vi "changetoStaging.vi"(7 "cmd":enum16{"off", "on", "undulator", "staging"}(ring), 8 "error in (no error)":errorcluster, 10 "send (true)":bool=TRUE) -> (0 "error out":errorcluster)   [LabVIEW 2013]
panel:
  in  "curent set":u16
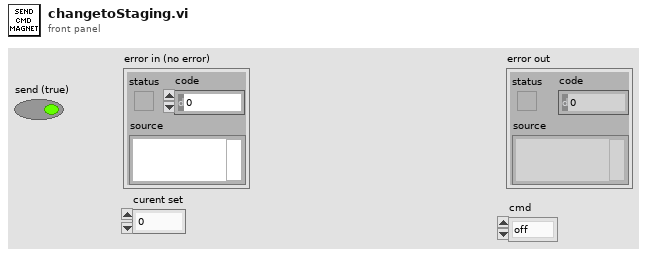
[diagram p1: front panel]
types:
  T1 = enum16{"Read", "Write", "ReadWrite", "BufferedRead", "BufferedReadWrite"}
  T2 = cluster{"data string":string, "data string":string, "data string":string, "data string":string}
  T3 = cluster{"match + rest of string":string, "match + rest of string":string, "data string":string, "data string":string}
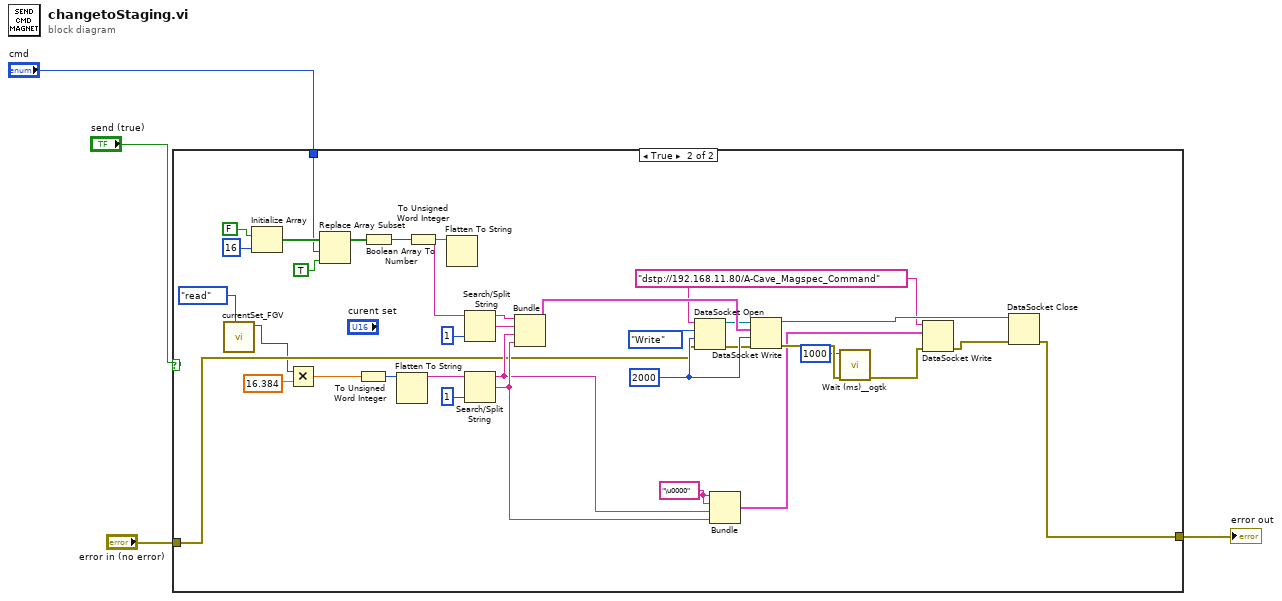
[diagram p0: block diagram]
diagram:
  n1 = case shown="True" "send (true)" {
    tunnel: "error in (no error)" -> [w5 w10]
    tunnel: [w5 w9] -> w2
    tunnel: "cmd" -> [_ w8]
    frame False {
    }
    frame True {
      w11 = "dstp://192.168.11.80/A-Cave_Magspec_Command" ("Target_URL")
      w21 = 2000 ("ms timeout (10000)")
      w22 = "\u0000" ("match + rest of string")
      n2 = call "currentSet_FGV.vi"("Enum"=enum16{"set", "read"}."read") -> ("curent set out"=w7:u16)  [unwired: 10 in]
      n3 = Initialize Array(FALSE, 16 ("dimension size")) -> (w39:bool[])
      n4 = Multiply(x=w7, y=16.384) -> (x*y=w28:dbl)
      n5 = Replace Array Subset(array=w39, new element=TRUE, index=w8) -> (w37:bool[])
      n6 = To Unsigned Word Integer(number=w28) -> (unsigned 16bit integer=w29:u16)
      n7 = Boolean Array To Number(Boolean array=w37) -> (number=w36:u32)
      n8 = Flatten To String(anything=w29) -> (data string=w30:string)  [unwired: 3 in, 2 out]
      n9 = To Unsigned Word Integer(number=w36) -> (unsigned 16bit integer=w26:u16)
      n10 = Flatten To String(anything=w26) -> (data string=w32:string)  [unwired: 3 in, 2 out]
      n11 = Search/Split String(string=w32, offset (0)=1) -> (substring before match=w34:string, match + rest of string=w35:string)  [unwired: 1 in, 1 out]
      n12 = Search/Split String(string=w30, offset (0)=1) -> (substring before match=w23:string, match + rest of string=w24:string)  [unwired: 1 in, 1 out]
      n13 = Bundle("data string"=w34, "data string"=w35, "data string"=w23, "data string"=w24) -> (w25:T2)  [unwired: 1 in]
      n14 = DataSocket Open(8:w10, 9:w21, 10:T1."Write" ("mode"), 11:w11) -> (0:w20:errorcluster, 3:w18:refnum<k13>)
      n15 = Bundle("match + rest of string"=w22, "match + rest of string"=w22, "data string"=w23, "data string"=w24) -> (w12:T3)  [unwired: 1 in]
      n16 = DataSocket Write(8:w20, 9:w21, 10:w25, 11:w18) -> (0:w16:errorcluster, 3:w19:refnum<k13>)  [unwired: 1 out]
      n17 = call <userlib>:"Wait (ms)__ogtk.vi"("error in (no error)"=w16, "milliseconds to wait"=u32 1000) -> ("error out"=w14:errorcluster)  [unwired: 8 in, 1 out]
      n18 = DataSocket Write(8:w14, 10:w12, 11:w11) -> (0:w13:errorcluster)  [unwired: 1 in, 2 out]
      n19 = DataSocket Close(8:w13, 11:w19) -> (0:w9:errorcluster)  [unwired: 1 in, 1 out]
    }
  }
  "error out" <- w2
